vi "Init Rx - Conversion Resources.vi"(8 "error in (no error)":errorcluster, 11 "Rx Loop Data":T1) -> (0 "error out":errorcluster, 3 "Rx Loop Data out":T1)   [LabVIEW 2019, in "UDP-Custom-Device Engine.lvlib"]
uses:
  UDP-Custom-Device Engine.lvlib
  Types/Engine - Rx Loop Data.ctl
  <vilib>/NI VeriStand/VeriStand Data/Byte Buffer/Byte Buffer.lvclass
  Types/Engine - General Resources.ctl
  <vilib>/NI VeriStand/VeriStand Data/Typedefs/Typedefs.Data Types.ctl
  Shared/Types/Shared - Duplex Settings.ctl
  Shared/Types/Shared - Header Details.ctl
  Shared/Types/Shared - Custom Header.ctl
  Types/Engine - Data Conversion Config.ctl
  <vilib>/NI VeriStand/VeriStand Data/Byte Buffer/Byte Buffer.Mapping.ctl
  Types/Engine - Rx Runtime Resources.ctl
  Types/Engine - Execution Config.ctl
  Shared/Types/Shared - Thread Management.ctl
  Types/Engine - Rx New Data Options Support.ctl
  Shared/Types/Shared - New Data Options.ctl
  Types/Engine - Rx Channel Refs.ctl
  <vilib>/NI/NIVS Inline Async API/_Data Access Engine/Data Access Engine/Types/Write.DVR.ctl
  <vilib>/NI/NIVS Inline Async API/_Data Access Engine/Access Type Classes/Write/Write.lvclass
  Types/Engine - Debug Resources.ctl
  <vilib>/NI VeriStand/VeriStand Data/Byte Buffer/Byte Buffer.Mapping.Create (Channel Pointer).vi
  <vilib>/NI VeriStand/VeriStand Data/Utilities/Utilities.Sizeof.Array.vi
  <vilib>/NI VeriStand/VeriStand Data/Utilities/Utilities.Sizeof.Scalar.vi
  <vilib>/NI VeriStand/VeriStand Data/VeriStand Data.lvlib
  <vilib>/NI/NIVS Inline Async API/_Data Access Engine/Data Access Engine/Data Access Engine.lvclass
  Shared/UDP-Custom-Device Shared.lvlib
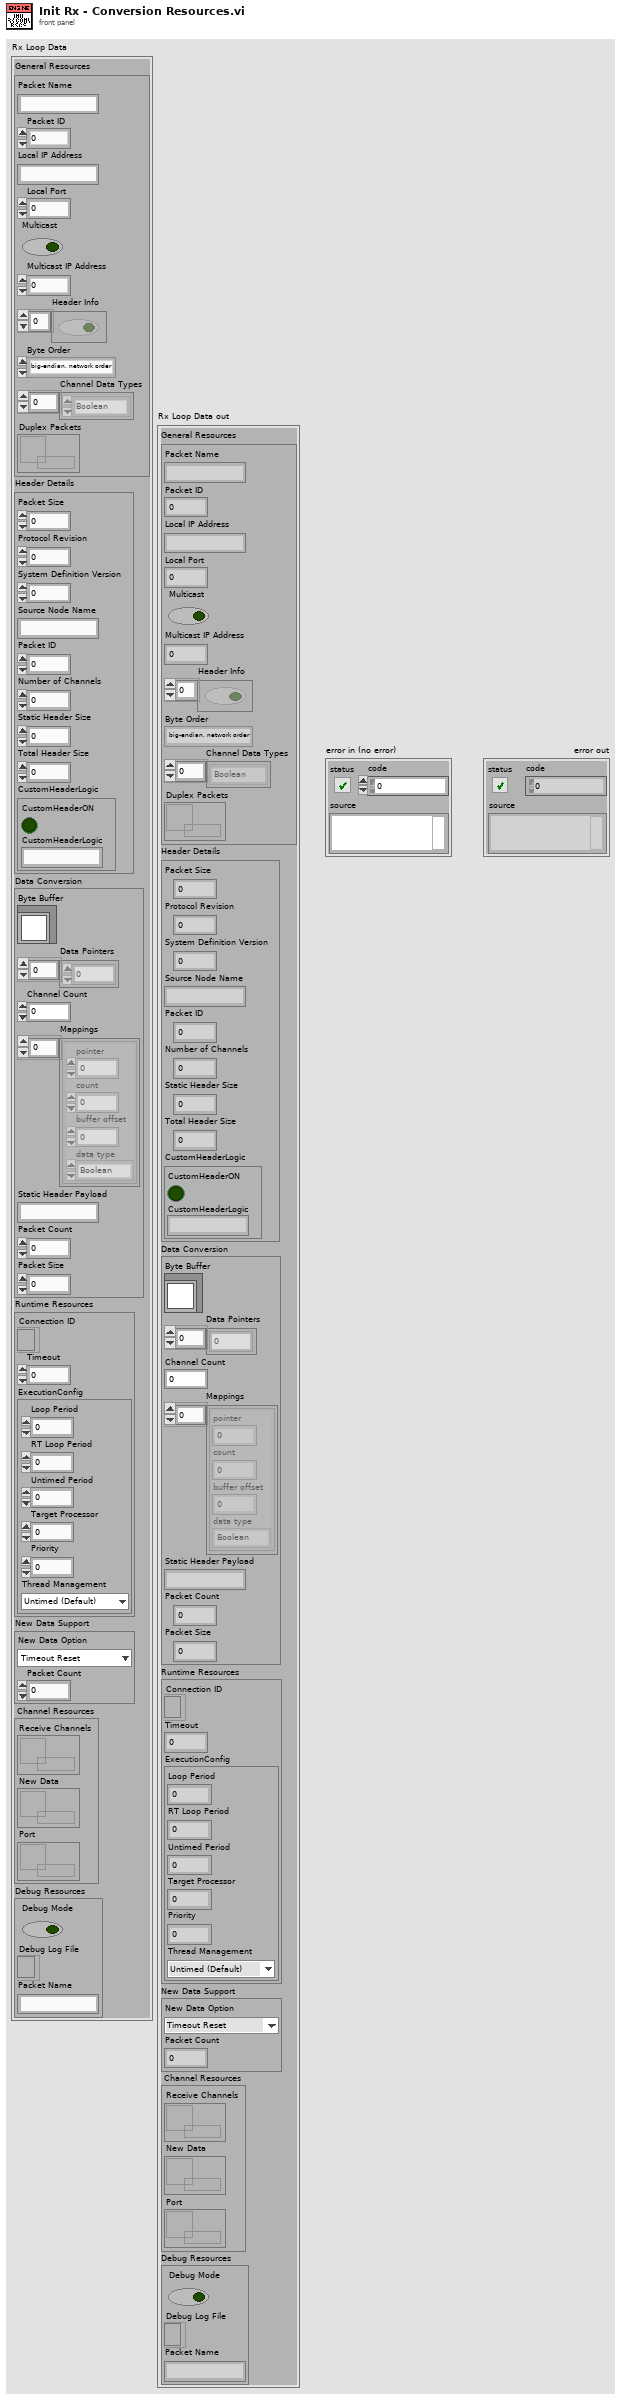
[diagram p1: front panel]
types:
  T1 = typedef "UDP-Custom-Device Engine.lvlib/Engine - Rx Loop Data.ctl" = cluster{"General Resources":T2, "Header Details":T4, "Data Conversion":T6, "Runtime Resources":T8, "New Data Support":T11, "Channel Resources":T13, "Debug Resources":T15}
  T2 = typedef "UDP-Custom-Device Engine.lvlib/Engine - General Resources.ctl" = cluster{"Packet Name":string, "Packet ID":i32, "Local IP Address":string, "Local Port":i32, "Multicast":bool, "Multicast IP Address":u32, "Header Info":bool[], "Byte Order":enum16{"big-endian, network order", "native, host order", "little-endian"}, "Channel Data Types":T3[], "Duplex Packets":refnum<data-value>}
  T3 = typedef "VeriStand Data.lvlib/Typedefs.Data Types.ctl" = enum16{"Boolean", "Single", "Double", "I8", "I16", "I32", "I64", "U8", "U16", "U32", "U64"}
  T4 = typedef "UDP-Custom-Device Shared.lvlib/Shared - Header Details.ctl" = cluster{"Packet Size":u16, "Protocol Revision":u8, "System Definition Version":u64, "Source Node Name":string, "Packet ID":u32, "Number of Channels":u32, "Static Header Size":u16, "Total Header Size":u16, "CustomHeaderLogic":T5}
  T5 = typedef "UDP-Custom-Device Shared.lvlib/Shared - Custom Header.ctl" = cluster{"CustomHeaderON":bool, "CustomHeaderLogic":string}
  T6 = typedef "UDP-Custom-Device Engine.lvlib/Engine - Data Conversion Config.ctl" = cluster{"Byte Buffer":refnum<class "Byte Buffer.lvclass">, "Data Pointers":u64[], "Channel Count":i32, "Mappings":T7[], "Static Header Payload":string, "Packet Count":dbl, "Packet Size":i32}
  T7 = typedef "VeriStand Data.lvlib/Byte Buffer.lvclass/Byte Buffer.Mapping.ctl" = cluster{"pointer":u64, "count":i64, "buffer offset":u64, "data type":T3}
  T8 = typedef "UDP-Custom-Device Engine.lvlib/Engine - Rx Runtime Resources.ctl" = cluster{"Connection ID":refnum<k16>, "Timeout":i32, "ExecutionConfig":T9}
  T9 = typedef "UDP-Custom-Device Engine.lvlib/Engine - Execution Config.ctl" = cluster{"Loop Period":i64, "RT Loop Period":i64, "Untimed Period":u32, "Target Processor":i32, "Priority":i32, "Thread Management":T10}
  T10 = typedef "UDP-Custom-Device Shared.lvlib/Shared - Thread Management.ctl" = enum16{"Untimed (Default)", "Timed (High Priority)"}
  T11 = typedef "UDP-Custom-Device Engine.lvlib/Engine - Rx New Data Options Support.ctl" = cluster{"New Data Option":T12, "Packet Count":dbl}
  T12 = typedef "UDP-Custom-Device Shared.lvlib/Shared - New Data Options.ctl" = enum16{"Timeout Reset", "Counter"}
  T13 = typedef "UDP-Custom-Device Engine.lvlib/Engine - Rx Channel Refs.ctl" = cluster{"Receive Channels":T14, "New Data":T14, "Port":T14}
  T14 = typedef "Data Access Engine.lvlib/Data Access Engine.lvclass/Write.DVR.ctl" = refnum<data-value>
  T15 = typedef "UDP-Custom-Device Engine.lvlib/Engine - Debug Resources.ctl" = cluster{"Debug Mode":bool, "Debug Log File":refnum<file>, "Packet Name":string}
  T16 = enum16{"big-endian, network order", "native, host order", "little-endian"}
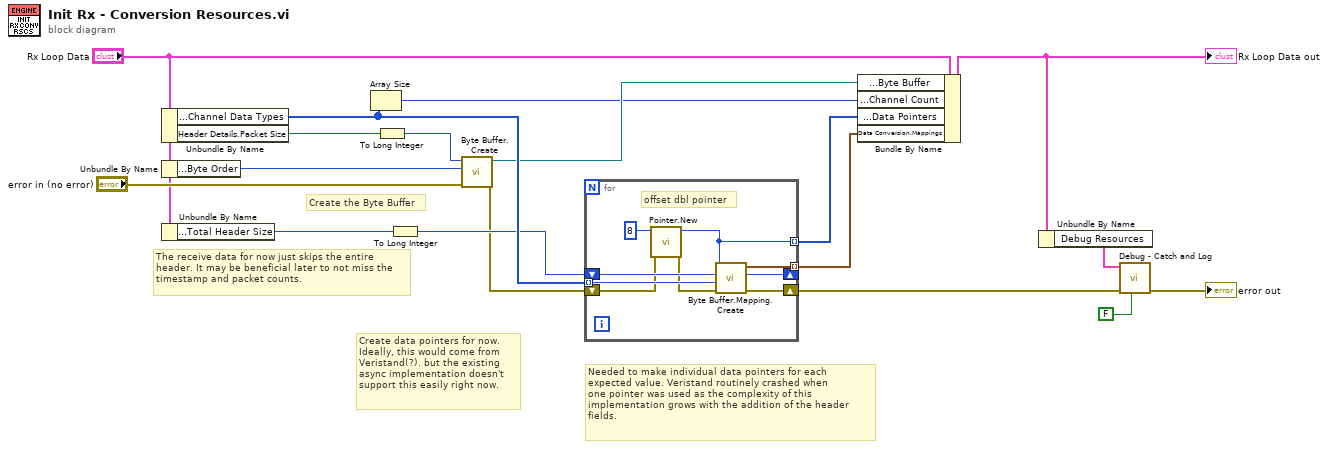
[diagram p0: block diagram]
diagram:
  # "Needed to make individual data pointers for each\nexpected value. Veristand routinely crashed when\none pointer was used as the complexity of this\nimplementation grows with the addition of the header\nfields."
  # "Create data pointers for now.\nIdeally, this would come from\nVeristand(?). but the existing\nasync implementation doesn't\nsupport this easily right now."
  # "The receive data for now just skips the entire\nheader. It may be beneficial later to not miss the\ntimestamp and packet counts."
  # "Create the Byte Buffer"
  n1 = Unbundle By Name("Rx Loop Data") -> ("General Resources.Channel Data Types"=w16:T3[], "Header Details.Packet Size"=w13:u16)
  n2 = Unbundle By Name("Rx Loop Data") -> ("General Resources.Byte Order"=w18:T16)
  n3 = Unbundle By Name("Rx Loop Data") -> ("Header Details.Total Header Size"=w10:u16)
  n4 = Array Size(array=w16) -> (size(s)=w8:i32)
  n5 = To Long Integer(number=w13) -> (32bit integer=w12:i32)
  n6 = To Long Integer(number=w10) -> (32bit integer=w9:i32)
  n7 = call <vilib>:"Byte Buffer.Create.vi"("error in (no error)"="error in (no error)", "byte order (big-endian)"=w18, "size"=w12) -> ("error out"=w7:errorcluster, "Byte Buffer"=w15:refnum<class "Byte Buffer.lvclass">)  [unwired: 7 in]
  n8 = for {
    tunnel: [w27] -> w14 mode=indexing
    tunnel: w16 -> [w25] mode=indexing
    shift-right: [w26] -> w3
    shift-left: w7 -> [w22]
    shift-right: [w24] -> _
    shift-left: w9 -> [w23]
    tunnel: [w19] -> w6 mode=indexing
    # "offset dbl pointer"
    n9 = call <vilib>:"Pointer.New.vi"("error in (no error)"=w22, "size in bytes"=8 ("x")) -> ("error out"=w21:errorcluster, "pointer"=w19:u64)  [unwired: 8 in]
    n10 = call-poly <vilib>:"Byte Buffer.Mapping.Create.vi"("error in (no error)"=w21, "data type"=w25, "buffer offset"=w23, "Channel Pointer"=w19) -> ("error out"=w26:errorcluster, "new buffer offset"=w24:u64, "mapping"=w27:T7)  [unwired: 5 in]
  }
  n11 = Bundle By Name(cluster="Rx Loop Data", "Data Conversion.Byte Buffer"=w15, "Data Conversion.Channel Count"=w8, "Data Conversion.Data Pointers"=w6, "Data Conversion.Mappings"=w14) -> (w1:T1)
  "Rx Loop Data out" <- w1
  n12 = Unbundle By Name(w1) -> ("Debug Resources"=w4:T15)
  n13 = call "Debug - Catch and Log.vi"("Clear Error?"=FALSE, "error in (no error)"=w3, "Debug Resources"=w4) -> ("error out"=→"error out":errorcluster)  [unwired: 8 in]
